vi "PCO_GetNumberOfImagesInSegment.vi"(8 "error in (no error)":errorcluster {"code" format="%x"}, 10 "wSegment":u16, 11 "ph":u64) -> (0 "error out":errorcluster {"code" format="%x"}, 1 "dwValidImageCnt":u32, 2 "ErrorMessage":i32 format="%x", 3 "ph out":u64, 5 "dwMaxImageCnt":u32)   [LabVIEW 2019, in "SDK.lvlib" / "ImageInformation.lvlib"]
doc: "<b>Description:</b>\nThis function returns the number of valid images and the maximum number of images within a distinct segment.\nWhile recording the number of valid images is dynamic - due to read and write accesses to the CamRAM. If the recording is stopped, the variable ValidImageCnt does not change anymore.\nIf the camera is in storage mode [recorder] the variable ValidImageCnt is counting up until the maximum image count is reached. After that the variable remains at the same value.\nIf the camera is in storage mode [FIFO buffer] the variable ValidImageCnt can decrease also, if the amount of transferred images is greater than the recorded images. If ValidImageCnt does stay at 1, transfer rate is equal or greater than recording rate. If ValidImageCnt is equal to maximum image count, the transfer rate is too slow and therefore recorded images are lost.\nIn storage mode [FIFO buffer] the ratio of valid number of images to the maximum number of images is a kind of filling level indicator.\n\n<b>Supported camera type:</b>\npco.dimax, pco.1200, pco.1600, pco.2000, pco.4000\n\n<b>Descriptor dependency:</b>\ndwGeneralCapsDESC1: NO_RECORDER"
uses:
  ImageInformation.lvlib
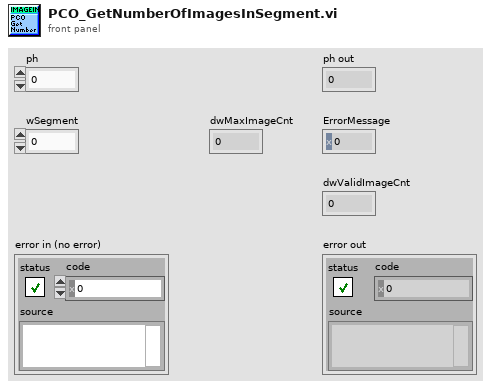
[diagram p1: front panel]
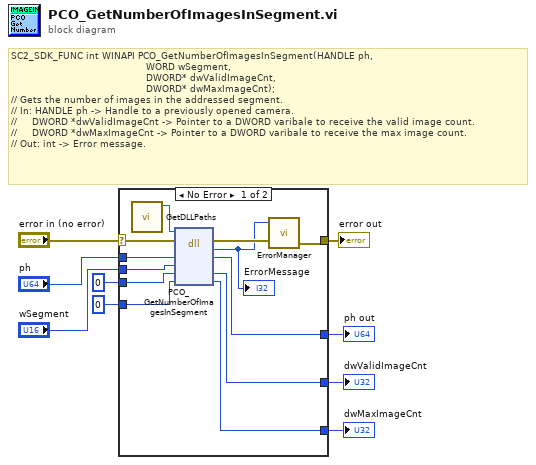
[diagram p0: block diagram]
diagram:
  # "SC2_SDK_FUNC int WINAPI PCO_GetNumberOfImagesInSegment(HANDLE ph, \n                                             WORD wSegment,\n                                             DWORD* dwValidImageCnt,\n                                             DWORD* dwMaxImageCnt);\n// Gets the number of images in the addressed segment.\n// In: HANDLE ph -> Handle to a previously opened camera.\n//     DWORD *dwValidImageCnt -> Pointer to a DWORD varibale to receive the valid image count.\n//     DWORD *dwMaxImageCnt -> Pointer to a DWORD varibale to receive the max image count.\n// Out: int -> Error message."
  n1 = case shown="No Error" "error in (no error)" {
    selector: "error in (no error)" -> [w14 w25]
    tunnel: "ph" -> [w21 w24]
    tunnel: [w20 w24] -> w8
    tunnel: "wSegment" -> [w19 _]
    tunnel: u32 0 ("dwValidImageCnt") -> [w18 w23]
    tunnel: [w17 w23] -> w5
    tunnel: u32 0 ("dwMaxImageCnt") -> [w16 w22]
    tunnel: [w15 w22] -> w3
    tunnel: [w12 w25] -> w2
    frame No Error {
      n2 = call "GetDLLPaths.vi"() -> ("SC2_Cam_Path"=w10:path)  [unwired: 8 in, 3 out]
      n3 = dll-call lib="?" fn="PCO_GetNumberOfImagesInSegment"(path in=w10, error in=w14, "ph"=w21, "wSegment"=w19, "dwValidImageCnt"=w18, "dwMaxImageCnt"=w16) -> (error out=w13:errorcluster, "return type"=w11:i32, "ph"=w20:u64, "dwValidImageCnt"=w17:u32, "dwMaxImageCnt"=w15:u32)  [unwired: 2 in, 1 out]
      "ErrorMessage" <- w11
      n4 = call "ErrorManager.vi"("error in (no error)"=w13, "error code"=w11) -> ("error out"=w12:errorcluster)  [unwired: 2 in, 1 out]
    }
    frame Error {
    }
  }
  "ph out" <- w8
  "dwValidImageCnt" <- w5
  "dwMaxImageCnt" <- w3
  "error out" <- w2
